vi "Begin.vi"(8 "error in":errorcluster) -> (0 "error out":errorcluster)   [LabVIEW 2015]
doc: "Called before other user functions, this VI is expected to open initial I/O refnums, load in file data, and do all program initialization. Notice that the <B>error out</B> terminal is simply used for data flow. Wiring it to other structures or subVIs ensures that this VI runs first."
uses:
  <vilib>/Rock Robotics/SystemInterfaces/DIO/FPGA_DIOPWMChannel.ctl
  <vilib>/Rock Robotics/WPI/DriverStation/WPI_DriverStationRobotMode2.ctl
  <vilib>/Rock Robotics/WPI/Joystick/WPI_JoystickDeviceEnum.ctl
  <vilib>/Rock Robotics/WPI/SafetyOutput/WPI_SafetyOutputConfigMenu.ctl
  <vilib>/Rock Robotics/WPI/Solenoid/WPI_SolenoidChannel.ctl
  <vilib>/Rock Robotics/SystemInterfaces/AI/FPGA_AIGyroChannel.ctl
  <vilib>/Rock Robotics/SystemInterfaces/DIO/FPGA_DIOChannel.ctl
  <vilib>/Rock Robotics/SystemInterfaces/AI/FPGA_AIChannel.ctl
  <vilib>/Rock Robotics/WPI/RobotDrive/WPI_RobotDriveOpen2MotorWithTalon.vi
  Robot Global Data.vi
  <vilib>/Rock Robotics/Network Tables/SD Write String Array.vi
  <vilib>/Rock Robotics/WPI/Solenoid/WPI_SolenoidOpenSingle.vi
  <vilib>/Rock Robotics/WPI/Gyro/WPI_GyroAnalogOpen.vi
  <vilib>/Rock Robotics/WPI/Counter/WPI_CounterDigitalInputToDigitalSource.vi
  <vilib>/Rock Robotics/WPI/Switch/WPI_SwitchOpenLimit.vi
  <vilib>/Rock Robotics/WPI/MotorControl/WPI_MotorControlOpen Talon.vi
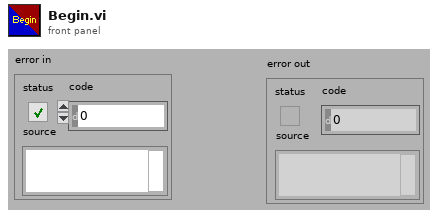
[diagram p1: front panel]
types:
  T1 = typedef "FPGA_AIChannel.ctl" = enum8{"AI 0", "AI 1", "AI 2", "AI 3", "AI MXP 0", "AI MXP 1", "AI MXP 2", "AI MXP 3", "Invalid"}
  T2 = typedef "WPI_SolenoidChannel.ctl" = enum8{"Solenoid 0", "Solenoid 1", "Solenoid 2", "Solenoid 3", "Solenoid 4", "Solenoid 5", "Solenoid 6", "Solenoid 7", "Invalid"}
  T3 = typedef "FPGA_DIOChannel.ctl" = enum8{"DIO 0", "DIO 1", "DIO 2", "DIO 3", "DIO 4", "DIO 5", "DIO 6", "DIO 7", "DIO 8", "DIO 9", "DIO MXP 0", "DIO MXP 1", "DIO MXP 2", "DIO MXP 3", "DIO MXP 4", "DIO MXP 5", "DIO MXP 6", "DIO MXP 7", "DIO MXP 8", "DIO MXP 9", "DIO MXP 10", "DIO MXP 11", "DIO MXP 12", "DIO MXP 13", "DIO MXP 14", "DIO MXP 15", "Invalid"}
  T4 = typedef "FPGA_AIGyroChannel.ctl" = enum8{"AI 0", "AI 1", "Invalid"}
  T5 = typedef "FPGA_DIOPWMChannel.ctl" = enum8{"PWM 0", "PWM 1", "PWM 2", "PWM 3", "PWM 4", "PWM 5", "PWM 6", "PWM 7", "PWM 8", "PWM 9", "PWM MXP 0", "PWM MXP 1", "PWM MXP 2", "PWM MXP 3", "PWM MXP 4", "PWM MXP 5", "PWM MXP 6", "PWM MXP 7", "PWM MXP 8", "PWM MXP 9", "Invalid"}
  T6 = typedef "WPI_JoystickDeviceEnum.ctl" = enum16{"USB 0", "USB 1", "USB 2", "USB 3", "USB 4", "USB 5"}
  T7 = typedef "WPI_SafetyOutputConfigMenu.ctl" = enum16{"Enable", "Disable"}
  T8 = typedef "WPI_DriverStationRobotMode2.ctl" = enum16{"Autonomous Disabled", "Autonomous Enabled", "Teleop Disabled", "Teleop Enabled", "Disconnected", "Finish", "Test Disabled", "Test Enabled", "Emergency Stopped"}
  T9 = typedef "WPI_JoystickDevRef.ctl" = cluster{"Device":T6}
  T10 = typedef "WPI_RobotDriveDevRef.ctl" = cluster{"DevStatus":errorcluster, "Motors[]":T11[], "Square Inputs":bool, "Max Output":dbl}
  T11 = typedef "WPI_MotorControlDeviceRef.ctl" = cluster{"DeviceStatus":errorcluster, "Type":T12, "PWM":cluster{"PWM Channel":T5, "DeadBand":T13}, "CAN":cluster{"Device Number":u8, "Control Mode":T14, "Semaphore":T15, "Max Vout":dbl, "TalonSRX Control Mode":T16}, "Invert":bool}
  T12 = typedef "WPI_MotorControlType.ctl" = enum16{"PWM", "CAN", "CANTalonSRX"}
  T13 = typedef "WPI_PWMDeadband.ctl" = cluster{"Name":string, "maxPositivePwm":i32, "minPositivePwm":i32, "centerPwm":i32, "maxNegativePwm":i32, "minNegativePwm":i32, "angularRange":u16}
  T14 = typedef "WPI_CANJaguar_ControlMode.ctl" = enum8{"Percent VBus", "Current", "Speed", "Position", "Voltage"}
  T15 = typedef "Semaphore RefNum" = refnum<k1>
  T16 = typedef "WPI_CANTalonSRX_APIControlMode.ctl" = enum8{"Percent VBus", "Speed", "Position", "Slave", "Unchanged / Invalid", "Voltage Compensation", "Current", "Motion Profile"}
  T17 = typedef "WPI_DigitalInputDevRef.ctl" = cluster{"DevStatus":errorcluster, "DIO Channel":T3}
  T18 = typedef "WPI_GyroDevRef.ctl" = cluster{"DevStatus":errorcluster, "Analog Channel":T1, "Offset":dbl, "Gain (VoltsPerDegree/Second)":dbl, "Gyro Type":enum16{"Analog", "XRS450"}, "Handle":i32, "SPI Bus":T19, "Device Found":bool, "Sample Rate":dbl, "Calibrate On Open":bool}
  T19 = typedef "spi_bus.ctl" = enum16{"SPI On-Board, CS0", "SPI On-Board, CS1", "SPI On-Board, CS2", "SPI On-Board, CS3", "SPI MXP", "Invalid"}
  T20 = typedef "WPI_SolenoidDevRef.ctl" = cluster{"DevStatus":errorcluster, "Pneumatics Control Module":u8, "Forward Solenoid Channel":T2, "Reverse Solenoid Channel":T2}
  T21 = typedef "FPGA_CounterEncoderSourceConvertionLVSourceType.ctl" = cluster{"DevStatus":errorcluster, "AnalogTriggerMode?":bool, "DigitalMode":cluster{"DIO Channel":T22}, "AnalogTriggerMode":cluster{"AnalogTriggerIndex":T23, "OutputType":T24}}
  T22 = typedef "FPGA_DIODigitalSourceChannel.ctl" = enum8{"DIO 0", "DIO 1", "DIO 2", "DIO 3", "DIO 4", "DIO 5", "DIO 6", "DIO 7", "DIO 8", "DIO 9", "DIO MXP 0", "DIO MXP 1", "DIO MXP 2", "DIO MXP 3", "DIO MXP 4", "DIO MXP 5", "DIO MXP 6", "DIO MXP 7", "DIO MXP 8", "DIO MXP 9", "DIO MXP 10", "DIO MXP 11", "DIO MXP 12", "DIO MXP 13", "DIO MXP 14", "DIO MXP 15", "Disabled"}
  T23 = typedef "FPGA_AnalogTriggerIndex.ctl" = enum8{"Trig 0", "Trig 1", "Trig 2", "Trig 3", "Trig 4", "Trig 5", "Trig 6", "Trig 7", "Invalid"}
  T24 = typedef "FPGA_AnalogTriggerOutType.ctl" = enum16{"InWindow", "TriggerState", "Rising", "Falling"}
  T25 = typedef "WPI_EncoderDevRef.ctl" = cluster{"DevStatus":errorcluster, "EncoderIndex":T26, "CounterIndex":T27, "DistancePerCount":dbl, "Decoding Type":T28}
  T26 = typedef "FPGA_EncoderIdx.ctl" = enum8{"Enc 0", "Enc 1", "Enc 2", "Enc 3", "Enc 4", "Enc 5", "Enc 6", "Enc 7", "Invalid"}
  T27 = typedef "FPGA_CounterCtrSystemIndex.ctl" = enum8{"Ctr 0", "Ctr 1", "Ctr 2", "Ctr 3", "Ctr 4", "Ctr 5", "Ctr 6", "Ctr 7", "Invalid"}
  T28 = typedef "WPI_EncoderType.ctl" = enum16{"1x", "2x", "4x"}
  T29 = typedef "WPI_PotentiometerDevRef.ctl" = cluster{"DevStatus":errorcluster, "Analog Channel":T1, "Invert Output":bool}
  T30 = typedef "WPI_SwitchDevRef.ctl" = cluster{"DevStatus":errorcluster, "DIO Channel":T3, "CntIndex":T27, "Normally Closed":bool}
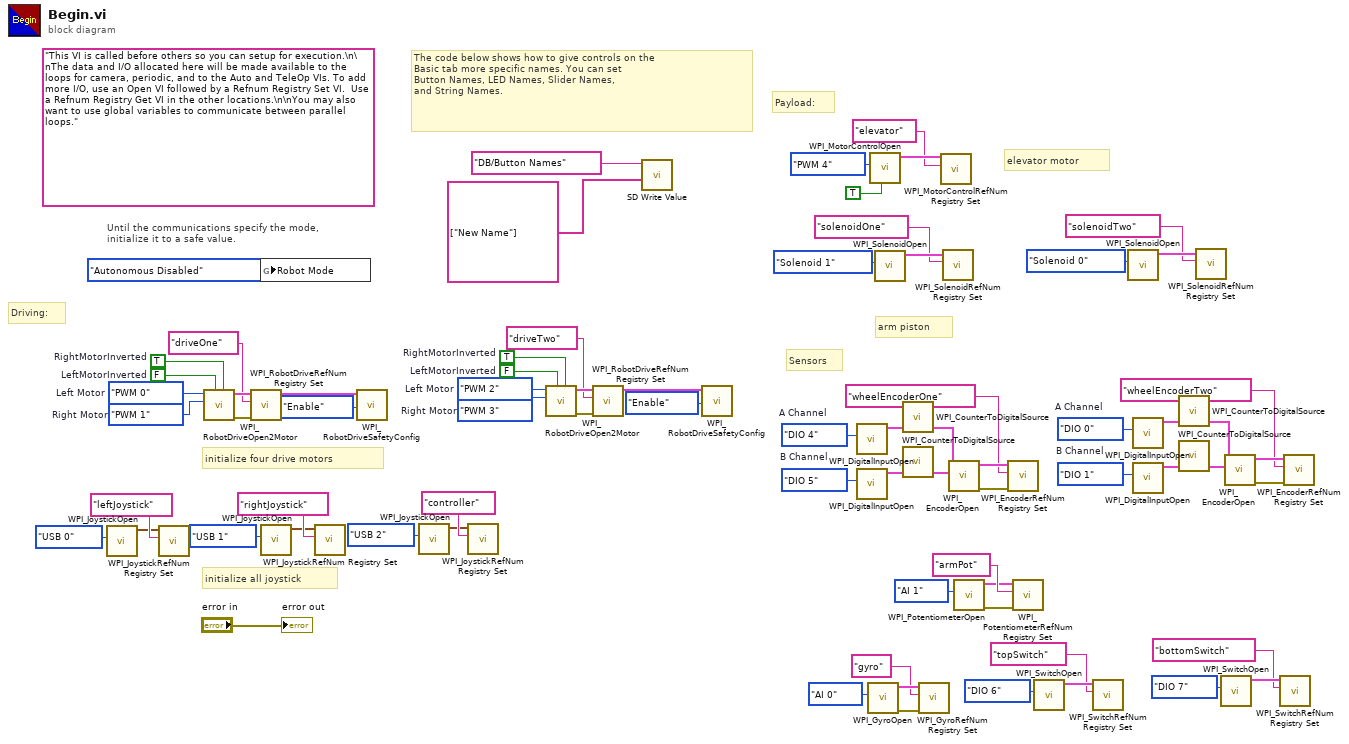
[diagram p0: block diagram]
diagram:
  w21 = FPGA_DIOChannel."DIO 1"  # B Channel
  w20 = FPGA_DIOChannel."DIO 0"  # A Channel
  w32 = FPGA_DIOChannel."DIO 5"  # B Channel
  w31 = FPGA_DIOChannel."DIO 4"  # A Channel
  w51 = FPGA_DIOPWMChannel."PWM 3"  # Right Motor
  w52 = FPGA_DIOPWMChannel."PWM 2"  # Left Motor
  w56 = FALSE  # LeftMotorInverted
  w57 = TRUE  # RightMotorInverted
  (unwired) "This VI is called before others so you can setup for execution.\n\nThe data and I/O allocated here will be made available to the loops for camera, periodic, and to the Auto and TeleOp VIs. To add more I/O, use an Open VI followed by a Refnum Registry Set VI.  Use a Refnum Registry Get VI in the other locations.\n\nYou may also want to use global variables to communicate between parallel loops."
  w67 = FPGA_DIOPWMChannel."PWM 1"  # Right Motor
  w68 = FPGA_DIOPWMChannel."PWM 0"  # Left Motor
  w72 = FALSE  # LeftMotorInverted
  w73 = TRUE  # RightMotorInverted
  # "arm piston"
  # "elevator motor"
  # "Sensors"
  # "Payload:"
  # "Driving:"
  # "The code below shows how to give controls on the\nBasic tab more specific names. You can set\nButton Names, LED Names, Slider Names,\nand String Names."
  # "initialize all joystick"
  # "Until the communications specify the mode,\ninitialize it to a safe value."
  # "initialize four drive motors"
  n1 = call <vilib>:"WPI_JoystickOpen.vi"("JoystickDevice"=WPI_JoystickDeviceEnum."USB 0") -> ("JoystickDevRef"=w62:T9)  [unwired: 10 in]
  n2 = call <vilib>:"WPI_JoystickRefNum Registry Set.vi"("refnum name"="leftJoystick", "JoystickDevRef"=w62) -> ()  [unwired: 8 in, 2 out]
  n3 = call-poly <vilib>:"WPI_RobotDriveOpen2Motor.vi"("Right Motor Inverted"=w73, "Left Motor Inverted"=w72, "Right Motor"=w67, "Left Motor"=w68) -> ("error out"=w69:errorcluster, "RobotDriveDevRef"=w71:T10)  [unwired: 1 in, 5 out]
  n4 = call <vilib>:"WPI_RobotDriveRefNum Registry Set.vi"("error in (no error)"=w69, "refnum name"="driveOne", "RobotDriveDevRef"=w71) -> ("RobotDriveDevRef"=w66:T10)  [unwired: 1 in, 7 out]
  n5 = global write "Robot Global Data.vi" "Robot Mode"(WPI_DriverStationRobotMode2."Autonomous Disabled" ("Robot Mode")) -> ()
  n6 = call <vilib>:"WPI_JoystickOpen.vi"("JoystickDevice"=WPI_JoystickDeviceEnum."USB 1") -> ("JoystickDevRef"=w47:T9)  [unwired: 10 in]
  n7 = call <vilib>:"WPI_JoystickRefNum Registry Set.vi"("refnum name"="rightJoystick", "JoystickDevRef"=w47) -> ()  [unwired: 8 in, 2 out]
  n8 = call <vilib>:"WPI_RobotDriveSafetyConfig.vi"("mode"=WPI_SafetyOutputConfigMenu."Enable", "RobotDriveDevRef"=w66) -> ()  [unwired: 8 in, 2 out]
  n9 = call <vilib>:"WPI_JoystickOpen.vi"("JoystickDevice"=WPI_JoystickDeviceEnum."USB 2") -> ("JoystickDevRef"=w44:T9)  [unwired: 10 in]
  n10 = call <vilib>:"WPI_JoystickRefNum Registry Set.vi"("refnum name"="controller", "JoystickDevRef"=w44) -> ()  [unwired: 8 in, 2 out]
  n11 = call-poly <vilib>:"WPI_RobotDriveOpen2Motor.vi"("Right Motor Inverted"=w57, "Left Motor Inverted"=w56, "Right Motor"=w51, "Left Motor"=w52) -> ("error out"=w53:errorcluster, "RobotDriveDevRef"=w55:T10)  [unwired: 1 in, 5 out]
  n12 = call <vilib>:"WPI_RobotDriveRefNum Registry Set.vi"("error in (no error)"=w53, "refnum name"="driveTwo", "RobotDriveDevRef"=w55) -> ("RobotDriveDevRef"=w50:T10)  [unwired: 1 in, 7 out]
  n13 = call-poly <vilib>:"SD Write Value.vi"("String Array"=string[] ["New Name"], "Name"="DB/Button Names") -> ()  [unwired: 8 in, 2 out]
  n14 = call <vilib>:"WPI_RobotDriveSafetyConfig.vi"("mode"=WPI_SafetyOutputConfigMenu."Enable", "RobotDriveDevRef"=w50) -> ()  [unwired: 8 in, 2 out]
  n15 = call <vilib>:"WPI_DigitalInputOpen.vi"("DIO Channel"=w31) -> ("DigitalInputDevRef"=w28:T17)  [unwired: 1 in, 9 out]
  n16 = call <vilib>:"WPI_DigitalInputOpen.vi"("DIO Channel"=w32) -> ("DigitalInputDevRef"=w29:T17)  [unwired: 1 in, 9 out]
  n17 = call-poly <vilib>:"WPI_GyroOpen.vi"("Analog Channel"=FPGA_AIGyroChannel."AI 0") -> ("error out"=w36:errorcluster, "GyroDevRef"=w35:T18)  [unwired: 8 in, 1 out]
  n18 = call-poly <vilib>:"WPI_MotorControlOpen.vi"("Invert"=TRUE, "PWM Channel"=FPGA_DIOPWMChannel."PWM 4") -> ("MotorControlDeviceRef"=w42:T11)  [unwired: 8 in, 1 out]
  n19 = call-poly <vilib>:"WPI_SolenoidOpen.vi"("Solenoid Channel"=WPI_SolenoidChannel."Solenoid 1") -> ("SolenoidDevRef"=w39:T20)  [unwired: 9 in, 1 out]
  n20 = call-poly <vilib>:"WPI_CounterToDigitalSource.vi"("DigitalInputDevRef"=w28) -> ("Digital Source"=w27:T21)  [unwired: 6 out]
  n21 = call-poly <vilib>:"WPI_CounterToDigitalSource.vi"("DigitalInputDevRef"=w29) -> ("Digital Source"=w30:T21)  [unwired: 6 out]
  n22 = call <vilib>:"WPI_GyroRefNum Registry Set.vi"("error in (no error)"=w36, "refnum name"="gyro", "GyroDevRef"=w35) -> ()  [unwired: 7 in, 2 out]
  n23 = call <vilib>:"WPI_MotorControlRefNum Registry Set.vi"("refnum name"="elevator", "MotorControlDevRef"=w42) -> ()  [unwired: 8 in, 2 out]
  n24 = call <vilib>:"WPI_SolenoidRefNum Registry Set.vi"("refnum name"="solenoidOne", "SolenoidDevRef"=w39) -> ()  [unwired: 8 in, 2 out]
  n25 = call <vilib>:"WPI_EncoderOpen.vi"("BSource"=w30, "ASource"=w27) -> ("error out"=w26:errorcluster, "EncoderDevRef"=w25:T25)  [unwired: 6 in, 2 out]
  n26 = call <vilib>:"WPI_PotentiometerOpen.vi"("Analog Channel"=FPGA_AIChannel."AI 1") -> ("error out"=w23:errorcluster, "PotDevRef"=w2:T29)  [unwired: 9 in]
  n27 = call <vilib>:"WPI_EncoderRefNum Registry Set.vi"("error in (no error)"=w26, "refnum name"="wheelEncoderOne", "EncoderDevRef"=w25) -> ()  [unwired: 7 in, 2 out]
  n28 = call <vilib>:"WPI_PotentiometerRefNum Registry Set.vi"("error in (no error)"=w23, "refnum name"="armPot", "PotDevRef"=w2) -> ()  [unwired: 7 in, 2 out]
  n29 = call-poly <vilib>:"WPI_SwitchOpen.vi"("DIO Channel"=FPGA_DIOChannel."DIO 6") -> ("SwitchDevRef"=w11:T30)  [unwired: 9 in, 1 out]
  n30 = call <vilib>:"WPI_SwitchRefNum Registry Set.vi"("refnum name"="topSwitch", "SwitchDevRef"=w11) -> ()  [unwired: 8 in, 2 out]
  n31 = call-poly <vilib>:"WPI_SolenoidOpen.vi"("Solenoid Channel"=WPI_SolenoidChannel."Solenoid 0") -> ("SolenoidDevRef"=w6:T20)  [unwired: 9 in, 1 out]
  n32 = call <vilib>:"WPI_DigitalInputOpen.vi"("DIO Channel"=w20) -> ("DigitalInputDevRef"=w17:T17)  [unwired: 1 in, 9 out]
  n33 = call <vilib>:"WPI_DigitalInputOpen.vi"("DIO Channel"=w21) -> ("DigitalInputDevRef"=w18:T17)  [unwired: 1 in, 9 out]
  n34 = call-poly <vilib>:"WPI_CounterToDigitalSource.vi"("DigitalInputDevRef"=w17) -> ("Digital Source"=w16:T21)  [unwired: 6 out]
  n35 = call-poly <vilib>:"WPI_CounterToDigitalSource.vi"("DigitalInputDevRef"=w18) -> ("Digital Source"=w19:T21)  [unwired: 6 out]
  n36 = call <vilib>:"WPI_SolenoidRefNum Registry Set.vi"("refnum name"="solenoidTwo", "SolenoidDevRef"=w6) -> ()  [unwired: 8 in, 2 out]
  n37 = call-poly <vilib>:"WPI_SwitchOpen.vi"("DIO Channel"=FPGA_DIOChannel."DIO 7") -> ("SwitchDevRef"=w8:T30)  [unwired: 9 in, 1 out]
  n38 = call <vilib>:"WPI_EncoderOpen.vi"("BSource"=w19, "ASource"=w16) -> ("error out"=w15:errorcluster, "EncoderDevRef"=w14:T25)  [unwired: 6 in, 2 out]
  n39 = call <vilib>:"WPI_SwitchRefNum Registry Set.vi"("refnum name"="bottomSwitch", "SwitchDevRef"=w8) -> ()  [unwired: 8 in, 2 out]
  n40 = call <vilib>:"WPI_EncoderRefNum Registry Set.vi"("error in (no error)"=w15, "refnum name"="wheelEncoderTwo", "EncoderDevRef"=w14) -> ()  [unwired: 7 in, 2 out]
  "error out" <- "error in"
